vi "settings handler.vi"(7 "Operation":enum16{"Open", "Write", "Read", "Close"}(ring), 8 "error in (no error)":errorcluster, 9 "Paths write":cluster{"Android":path, "Version":path}, 11 "Write":T1={"COM"="", "baud rate"=115200, "data bits"=8, "parity"=enum."None", "stop bits"=10, "flow control"=enum."None", "delay"=50} {"stop bits" items=["1.0"=10, "1.5"=15, "2.0"=20]; "baud rate" max=921600; "data bits" max=16}) -> (0 "Error Out":errorcluster, 1 "Paths read":cluster{"Android":path, "Version":path}, 3 "Read":T1={"COM"="", "baud rate"=115200, "data bits"=8, "parity"=enum."None", "stop bits"=10, "flow control"=enum."None", "delay"=50} {"stop bits" items=["1.0"=10, "1.5"=15, "2.0"=20]; "baud rate" max=921600; "data bits" max=16})   [LabVIEW 2021]
uses:
  <vilib>/Utility/config.llb/Write Key (String).vi
  <vilib>/Utility/config.llb/Read Key (String).vi
  <vilib>/Utility/config.llb/NI_LVConfig.lvlib
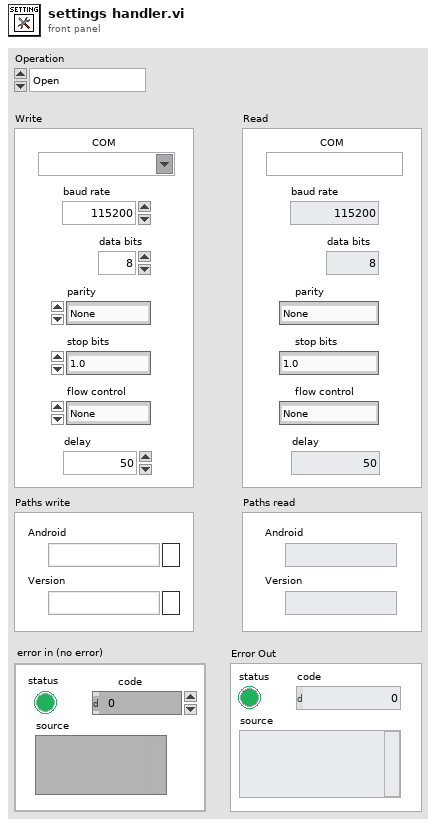
[diagram p1: front panel]
types:
  T1 = cluster{"COM":refnum<visa-resource-name>, "baud rate":u32, "data bits":u8, "parity":enum16{"None", "Odd", "Even", "Mark", "Space"}, "stop bits":u16, "flow control":enum16{"None", "XON/XOFF", "RTS/CTS", "DTR/DSR"}, "delay":u16}
  T2 = typedef "NI_LVConfig.lvlib/Config Data RefNum.ctl" = refnum<k1>
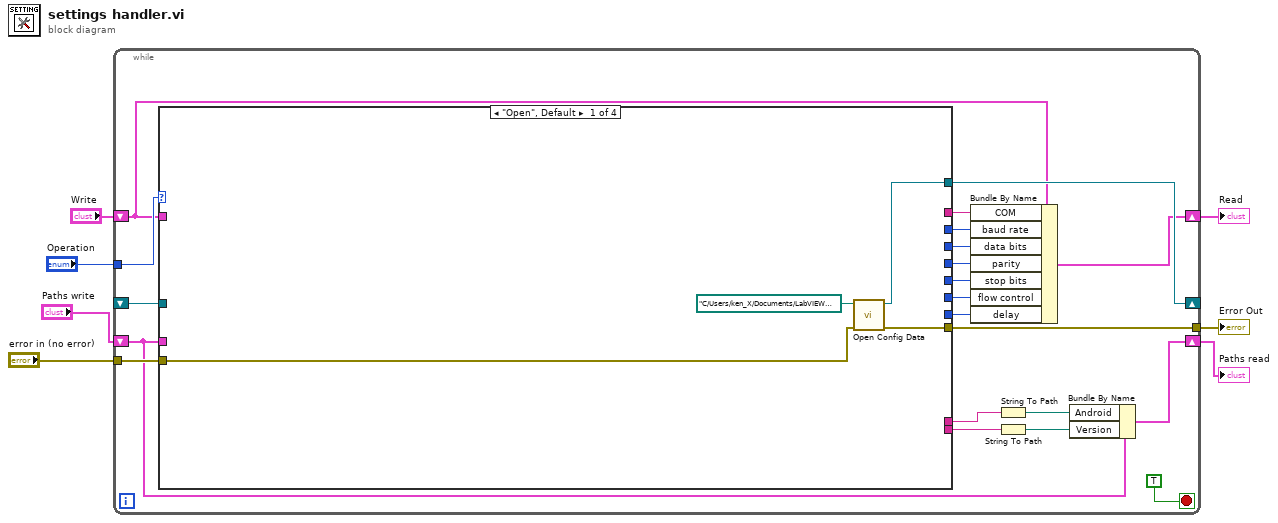
[diagram p0: block diagram]
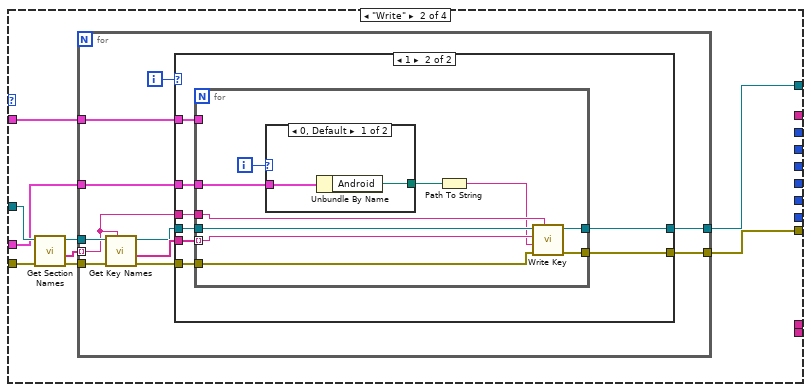
[diagram p2: hidden frame]
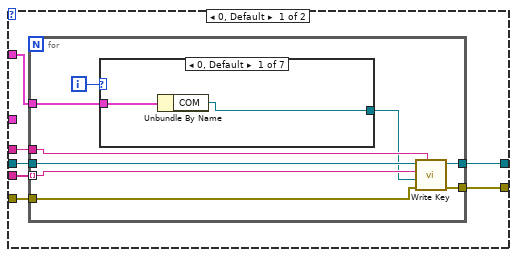
[diagram p3: hidden frame]
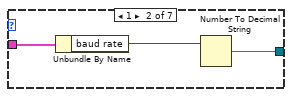
[diagram p4: hidden frame]
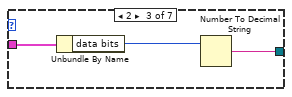
[diagram p5: hidden frame]
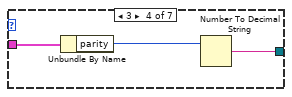
[diagram p6: hidden frame]
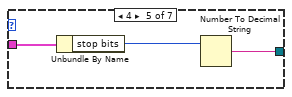
[diagram p7: hidden frame]
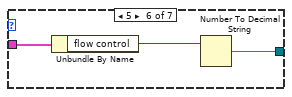
[diagram p8: hidden frame]
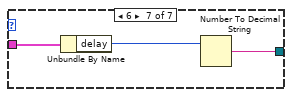
[diagram p9: hidden frame]
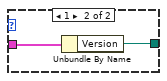
[diagram p10: hidden frame]
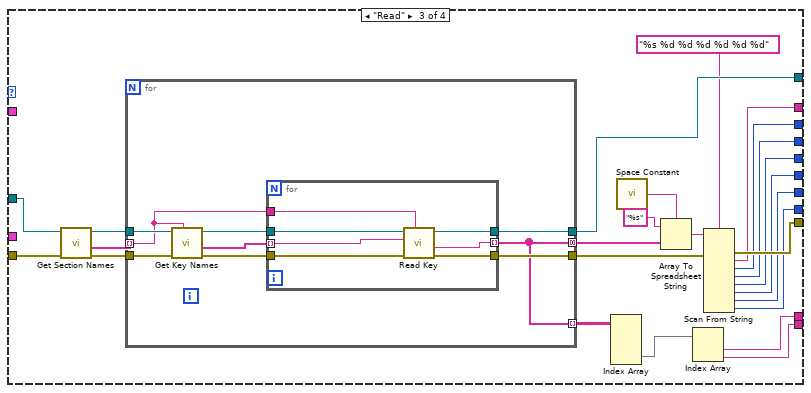
[diagram p11: hidden frame]
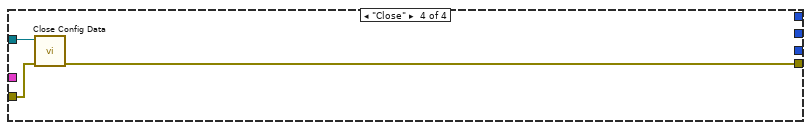
[diagram p12: hidden frame]
diagram:
  n1 = while {
    tunnel: "error in (no error)" -> [w28]
    tunnel: [w27] -> w6
    shift-right: [w26] -> _
    shift-left: _ -> [w24]
    shift-right: [w21] -> w3
    shift-left: "Write" -> [w22]
    tunnel: "Operation" -> [w23]
    shift-right: [w12] -> w1
    shift-left: "Paths write" -> [w13]
    stop <- TRUE stop-if-true
    n2 = case shown="\"Open\", Default" w23 {
      tunnel: w28 -> [w31 w38 w133 w153]
      tunnel: [w30 w34 w123 w152] -> w27
      tunnel: [w29 w35 w129 _] -> w26
      tunnel: w24 -> [_ w37 w134 w151]
      tunnel: [_ _ w120 _] -> w20
      tunnel: [_ _ w119 _] -> w19
      tunnel: [_ _ w118 _] -> w18
      tunnel: [_ _ w117 _] -> w17
      tunnel: [_ _ w116 _] -> w16
      tunnel: w22 -> [_ w36 _ _]
      tunnel: [_ _ w115 _] -> w15
      tunnel: [_ _ w121 _] -> w14
      tunnel: w13 -> [_ w33 _ _]
      tunnel: [_ _ w112 _] -> w9
      tunnel: [_ _ w111 _] -> w8
      frame "Open", Default {
        n3 = call <vilib>:"Open Config Data.vi"("error in (no error)"=w31, "configuration file path"=path "C:/Users/ken_X/Documents/LabVIEW projects/Project-B/settings/settings.ini" ("file path (use dialog)")) -> ("error out"=w30:errorcluster, "refnum"=w29:T2)  [unwired: 7 in, 1 out]
      }
      frame "Write" {
        n4 = call <vilib>:"Get Section Names.vi"("error in (no error)"=w38, "refnum"=w37) -> ("error out"=w39:errorcluster, "section names"=w41:string[], "refnum out"=w40:T2)  [unwired: 7 in]
        n5 = for {
          tunnel: w41 -> [w50] mode=indexing
          tunnel: w40 -> [w52]
          tunnel: w39 -> [w51]
          tunnel: [w46] -> w35
          tunnel: [w45] -> w34
          tunnel: w36 -> [w44]
          tunnel: w33 -> [w42]
          i -> [w43]
          n6 = call <vilib>:"Get Key Names.vi"("section"=w50, "error in (no error)"=w51, "refnum"=w52) -> ("error out"=w47:errorcluster, "key names"=w49:string[], "refnum out"=w48:T2)  [unwired: 5 in, 1 out]
          n7 = case shown="1" w43 {
            tunnel: w50 -> [w59 w96]
            tunnel: w49 -> [w58 w95]
            tunnel: w48 -> [w57 w94]
            tunnel: w47 -> [w56 w93]
            tunnel: [w55 w92] -> w46
            tunnel: [w54 w91] -> w45
            tunnel: w44 -> [w53 w90]
            tunnel: w42 -> [_ w89]
            frame 0, Default {
              n8 = for {
                tunnel: w59 -> [w68]
                tunnel: w58 -> [w67] mode=indexing
                tunnel: w57 -> [w66]
                tunnel: w56 -> [w65]
                tunnel: [w64] -> w55
                tunnel: [w63] -> w54
                tunnel: w53 -> [w61]
                i -> [w62]
                n9 = case shown="0, Default" w62 {
                  tunnel: w61 -> [w70 w73 w76 w79 w82 w85 w88]
                  tunnel: [w69 w71 w74 w78 w80 w84 w87] -> w60
                  frame 0, Default {
                    n10 = Unbundle By Name(w70) -> ("COM"=w69:refnum<visa-resource-name>)
                  }
                  frame 1 {
                    n11 = Unbundle By Name(w73) -> ("baud rate"=w72:u32)
                    n12 = Number To Decimal String(number=w72) -> (decimal integer string=w71:string)  [unwired: 1 in]
                  }
                  frame 2 {
                    n13 = Unbundle By Name(w76) -> ("data bits"=w75:u8)
                    n14 = Number To Decimal String(number=w75) -> (decimal integer string=w74:string)  [unwired: 1 in]
                  }
                  frame 3 {
                    n15 = Unbundle By Name(w79) -> ("parity"=w77:enum16{"None", "Odd", "Even", "Mark", "Space"})
                    n16 = Number To Decimal String(number=w77) -> (decimal integer string=w78:string)  [unwired: 1 in]
                  }
                  frame 4 {
                    n17 = Unbundle By Name(w82) -> ("stop bits"=w81:u16)
                    n18 = Number To Decimal String(number=w81) -> (decimal integer string=w80:string)  [unwired: 1 in]
                  }
                  frame 5 {
                    n19 = Unbundle By Name(w85) -> ("flow control"=w83:enum16{"None", "XON/XOFF", "RTS/CTS", "DTR/DSR"})
                    n20 = Number To Decimal String(number=w83) -> (decimal integer string=w84:string)  [unwired: 1 in]
                  }
                  frame 6 {
                    n21 = Unbundle By Name(w88) -> ("delay"=w86:u16)
                    n22 = Number To Decimal String(number=w86) -> (decimal integer string=w87:string)  [unwired: 1 in]
                  }
                }
                n23 = call-poly <vilib>:"Write Key.vi"("section"=w68, "error in (no error)"=w65, "value"=w60, "key"=w67, "refnum"=w66) -> ("error out"=w63:errorcluster, "refnum out"=w64:T2)  [unwired: 4 in, 1 out]
              }
            }
            frame 1 {
              n24 = for {
                tunnel: w96 -> [w106]
                tunnel: w95 -> [w105] mode=indexing
                tunnel: w94 -> [w104]
                tunnel: w93 -> [w103]
                tunnel: [w102] -> w92
                tunnel: [w101] -> w91
                tunnel: w90 -> [_]
                tunnel: w89 -> [w99]
                i -> [w100]
                n25 = case shown="0, Default" w100 {
                  tunnel: w99 -> [w107 w110]
                  tunnel: [w108 w109] -> w98
                  frame 0, Default {
                    n26 = Unbundle By Name(w107) -> ("Android"=w108:path)
                  }
                  frame 1 {
                    n27 = Unbundle By Name(w110) -> ("Version"=w109:path)
                  }
                }
                n28 = Path To String(path=w98) -> (string=w97:string)
                n29 = call-poly <vilib>:"Write Key.vi"("section"=w106, "error in (no error)"=w103, "value"=w97, "key"=w105, "refnum"=w104) -> ("error out"=w101:errorcluster, "refnum out"=w102:T2)  [unwired: 4 in, 1 out]
              }
            }
          }
        }
      }
      frame "Read" {
        n30 = call <vilib>:"Get Section Names.vi"("error in (no error)"=w133, "refnum"=w134) -> ("error out"=w130:errorcluster, "section names"=w132:string[], "refnum out"=w131:T2)  [unwired: 7 in]
        n31 = for {
          tunnel: w132 -> [w141] mode=indexing
          tunnel: w131 -> [w143]
          tunnel: w130 -> [w142]
          tunnel: [w137] -> w129
          tunnel: [w136] -> w124
          tunnel: [w135] -> w127 mode=concatenating
          tunnel: [w135] -> w114 mode=indexing
          n32 = call <vilib>:"Get Key Names.vi"("section"=w141, "error in (no error)"=w142, "refnum"=w143) -> ("error out"=w138:errorcluster, "key names"=w140:string[], "refnum out"=w139:T2)  [unwired: 5 in, 1 out]
          n33 = for {
            tunnel: w141 -> [w150]
            tunnel: w140 -> [w149] mode=indexing
            tunnel: w139 -> [w148]
            tunnel: w138 -> [w147]
            tunnel: [w146] -> w137
            tunnel: [w145] -> w136
            tunnel: [w144] -> w135 mode=indexing
            n34 = call-poly <vilib>:"Read Key.vi"("section"=w150, "error in (no error)"=w147, "key"=w149, "refnum"=w148) -> ("error out"=w145:errorcluster, "value"=w144:string, "refnum out"=w146:T2)  [unwired: 4 in, 1 out]
          }
        }
        n35 = Index Array(array=w114) -> (element #2=w113:string[])  [unwired: 4 in, 1 out]
        n36 = call <vilib>:"Space Constant.vi"() -> ("String"=w122:string)
        n37 = Array To Spreadsheet String(delimiter (Tab)=w122, array=w127, 3:"%s" ("format string")) -> (spreadsheet string=w125:string)
        n38 = Index Array(array=w113) -> (element #1=w112:string, element #2=w111:string)  [unwired: 2 in]
        n39 = Scan From String(format string="%s %d %d %d %d %d %d", input string=w125, error in=w124) -> (error out=w123:errorcluster, output 1=w121:string, output 2=w120:i32, output 3=w119:i32, output 4=w118:i32, output 5=w117:i32, output 6=w116:i32, output 7=w115:i32)  [unwired: 8 in, 2 out]
      }
      frame "Close" {
        n40 = call <vilib>:"Close Config Data.vi"("error in (no error)"=w153, "refnum"=w151) -> ("error out"=w152:errorcluster)  [unwired: 8 in, 1 out]
      }
    }
    n41 = Bundle By Name(cluster=w22, "COM"=w14, "baud rate"=w20, "data bits"=w19, "parity"=w18, "stop bits"=w17, "flow control"=w16, "delay"=w15) -> (w21:T1)
    n42 = String To Path(string=w9) -> (path=w11:path)
    n43 = String To Path(string=w8) -> (path=w10:path)
    n44 = Bundle By Name(cluster=w13, "Android"=w11, "Version"=w10) -> (w12:cluster{"Android":path, "Version":path})
  }
  "Error Out" <- w6
  "Read" <- w3
  "Paths read" <- w1
